vi "LV to ITX XY AutoPlot.vi"(4 "X,Y Log":i32[](array[numeric]), 6 "X,Y Labels":string[](array[string])=["x label", "y label"], 7 "Notes":string, 8 "error in":errorcluster, 10 "XY-Data []":cluster{"X  array":dbl[], "Y  Array":dbl[]}[](array[cluster]), 11 "path":path=path "C:/Users/voodoo.SEAGATE/Desktop/datatest") -> (0 "error out":errorcluster, 3 "file":path=path "C:/Users/voodoo.SEAGATE/Desktop/datatest/datatest.000019.itx")   [LabVIEW 2019, in "LV-Data.ITX.lvclass"]
doc: "Write your XY data to ITX file. This AutoPlot VI adds commands to automatically create a graph in Igor to quickly view your data.\n\n-- path: base path to save data\n-- filename: base filename\n-- Notes: add any notes here to help you remember what experiment you did\n-- XY Array: Array of Clusters (ie, Array of XY graphs)\n-- wavenames: Give each data array a unique name such as \"time, bias, current,...\"\n-- X,Y Labels: For plotting in Igor. Can be ignored.\n-- X,Y Log: Do you wan to show X or Y on Log scale in Igor?"
uses:
  LV-Data.ITX.lvclass
  ITX Commands/ITX Commands.lvclass
  LV-Data/LV-Data.lvclass
  LV-Data/Typedefs/Operation--enum.ctl
  LV-Data/Typedefs/File Type--enum.ctl
  4e7104cf-761e-49f4-a8a0-3f14be840846.vi
panel:
  # "Below are relevant for creating graphs in Igor"
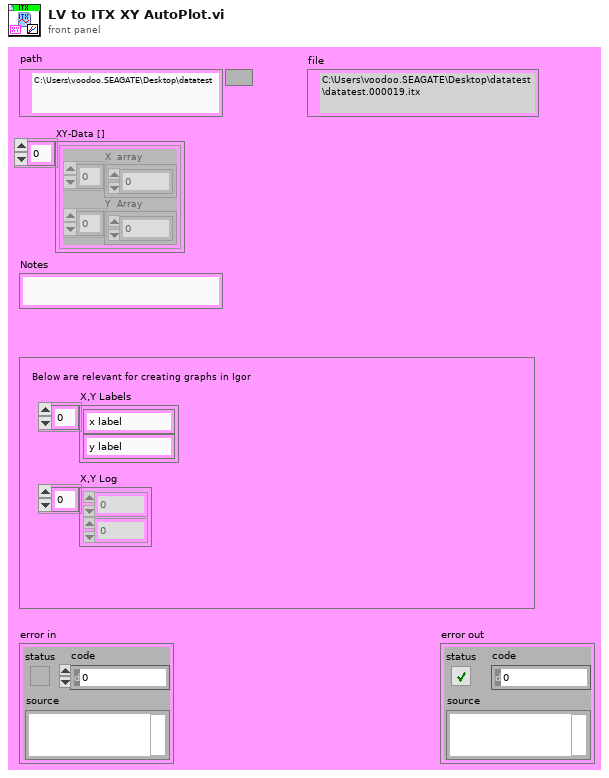
[diagram p1: front panel]
types:
  T1 = typedef "LV-Data.lvclass/File Type--enum.ctl" = enum16{"DAT", "ITX", "TDMS", "VI"}
  T2 = typedef "LV-Data.lvclass/Operation--enum.ctl" = enum16{"Read", "Write", "Write + Append"}
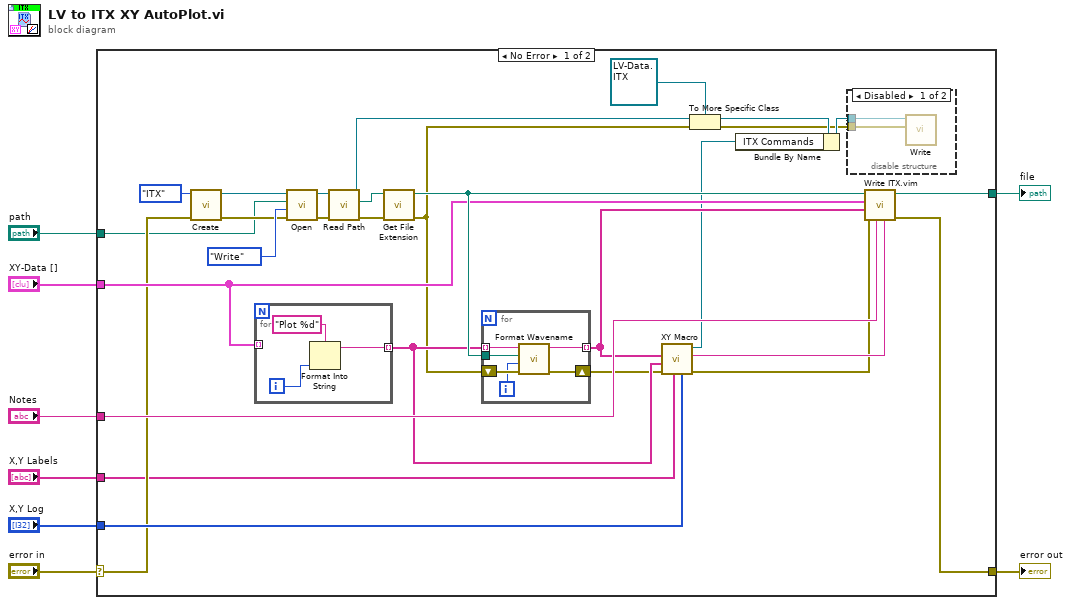
[diagram p0: block diagram]
diagram:
  n1 = case shown="No Error" "error in" {
    selector: "error in" -> [w23 w50]
    tunnel: "path" -> [w21 w49]
    tunnel: "X,Y Labels" -> [w18 _]
    tunnel: [w37 w49] -> w6
    tunnel: "X,Y Log" -> [w36 _]
    tunnel: "XY-Data []" -> [w27 _]
    tunnel: [w35 w50] -> w2
    tunnel: "Notes" -> [w33 _]
    frame No Error {
      n2 = call "Create.vi"("error in (no error)"=w23, "File Type"=File_Type--enum."ITX") -> ("error out"=w22:errorcluster, "Data out"=w24:refnum<class "LV-Data.lvclass">)  [unwired: 8 in]
      n3 = for {
        tunnel: w27 -> [_] mode=indexing
        tunnel: [w38] -> w19 mode=indexing
        i -> [w40]
        n4 = Format Into String(format string="Plot %d", w40) -> (resulting string=w38:string)  [unwired: 2 in, 1 out]
      }
      n5 = call-dynamic "Open.vi"("error in (no error)"=w22, "Operation"=Operation--enum."Write", "Path"=w21, "Data in"=w24) -> ("error out"=w28:errorcluster, "Data out"=w29:refnum<class "LV-Data.lvclass">)  [unwired: 6 in]
      n6 = call "Read Path.vi"("error in (no error)"=w28, "Data Save"=w29) -> ("error out"=w31:errorcluster, "Path"=w32:path, "Data Save out"=w15:refnum<class "LV-Data.lvclass">)  [unwired: 7 in]
      n7 = call <vilib>:"Get File Extension.vi"("error in (no error)"=w31, "file"=w32) -> ("error out"=w9:errorcluster, "dup file"=w30:path)  [unwired: 5 in, 3 out]
      n8 = for {
        tunnel: w19 -> [w46] mode=indexing
        shift-right: [w44] -> w17
        shift-left: w9 -> [w45]
        tunnel: [w43] -> w20 mode=indexing
        tunnel: w30 -> [w41]
        i -> [w42]
        n9 = call "Format Wavename.vi"("error in (no error)"=w45, "Index"=w42, "Path"=w41, "Name"=w46) -> ("error out"=w44:errorcluster, "Formatted wavename"=w43:string)  [unwired: 6 in]
      }
      n10 = call "XY Macro.vi"("X,Y Log"=w36, "X,Y Labels"=w18, "error in (no error)"=w17, "Plot labels"=w19, "wavenames"=w20) -> ("error out"=w16:errorcluster, "Commands"=w34:string, "ITX Commands out"=w13:refnum<class "ITX Commands.lvclass">)  [unwired: 4 in]
      n11 = To More Specific Class(target class=refnum<class "LV-Data.ITX.lvclass"> refnum ("LV-Data.ITX.lvclass"), reference=w15, error in=w9) -> (specific class reference=w12:refnum<class "LV-Data.ITX.lvclass">, error out=w10:errorcluster)
      n12 = Bundle By Name(cluster=w12, "ITX Commands"=w13) -> (w11:refnum<class "LV-Data.ITX.lvclass">)
      n13 = disable-structure shown="Disabled" {
        disable-tunnel: w11 -> [w48 _]
        disable-tunnel: w10 -> [w47 _]
        frame Disabled {
          n14 = call-dynamic "Write.vi"("error in (no error)"=w47, "Data.ITX in"=w48) -> ()  [unwired: 7 in, 3 out]
        }
        frame Enabled {
        }
      }
      n15 = call "Write ITX.vim"("commands"=w34, "notes"=w33, "error in"=w16, "wavename"=w20, "values"=w27, "filename"=w30) -> ("error out"=w35:errorcluster, "filename out"=w37:path)  [unwired: 3 in, 1 out]
    }
    frame Error {
    }
  }
  "file" <- w6
  "error out" <- w2
